vi "downloadpcx.vi"(8 "error in (no error)":errorcluster caption="entrée d'erreur (pas d'erreur)", 10 "image_name":string, 11 "filename":string) -> (0 "error out":errorcluster caption="sortie d'erreur", 1 "function return":i32, 2 "image_name out":string, 3 "filename out":string)   [LabVIEW 2020, in "Library Instrument & Equipement.lvlib" / "Library Printer.lvlib" / "TSCLIB.lvlib"]
doc: "EXPORT int CALLBACK downloadpcx (char *filename,char *image_name);"
uses:
  TSCLIB.lvlib
  TSCLIB.dll
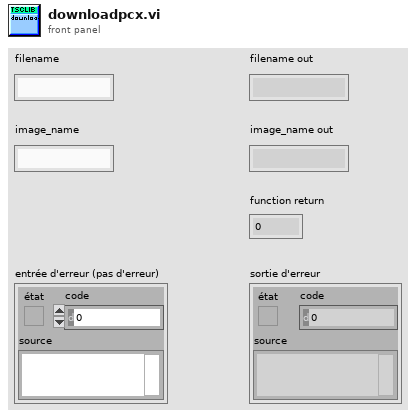
[diagram p1: front panel]
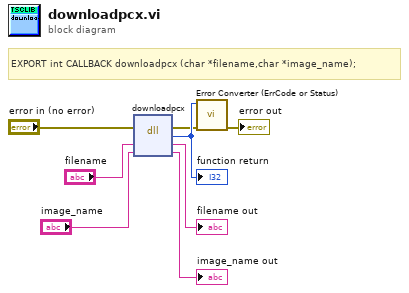
[diagram p0: block diagram]
diagram:
  # "EXPORT int CALLBACK downloadpcx (char *filename,char *image_name);"
  n1 = dll-call lib="C:/Users/ngarcin/OneDrive - Altyor/Standard TB/Class/Printer/Printer TSC/TSCLIB/TSCLIB.dll" fn="downloadpcx"(error in="error in (no error)", "filename"="filename", "image_name"="image_name") -> (error out=w2:errorcluster, "type de retour"=w8:i32, "filename"=→"filename out":string, "image_name"=→"image_name out":string)  [unwired: 2 in, 1 out]
  "function return" <- w8
  n2 = call "Error Converter (ErrCode or Status).vi"("error in (no error)"=w2, "error code"=w8) -> ("error out"=→"error out":errorcluster)  [unwired: 9 in]
